vi "WT-Logger.vi"() -> ()   [LabVIEW 2017]
uses:
  <vilib>/Utility/file.llb/Write Delimited Spreadsheet (string).vi
  <vilib>/Utility/file.llb/Write Delimited Spreadsheet (DBL).vi
panel:
  out "Heart Beat":bool
  in  "File Output?":bool
  in  "Log_Data":bool
  out "MWTP":dbl(graph)
  out "LATP":dbl(graph)
  out "LATT":dbl(graph)
  out "LATD":dbl(graph)
  out "MWTV":dbl(graph)
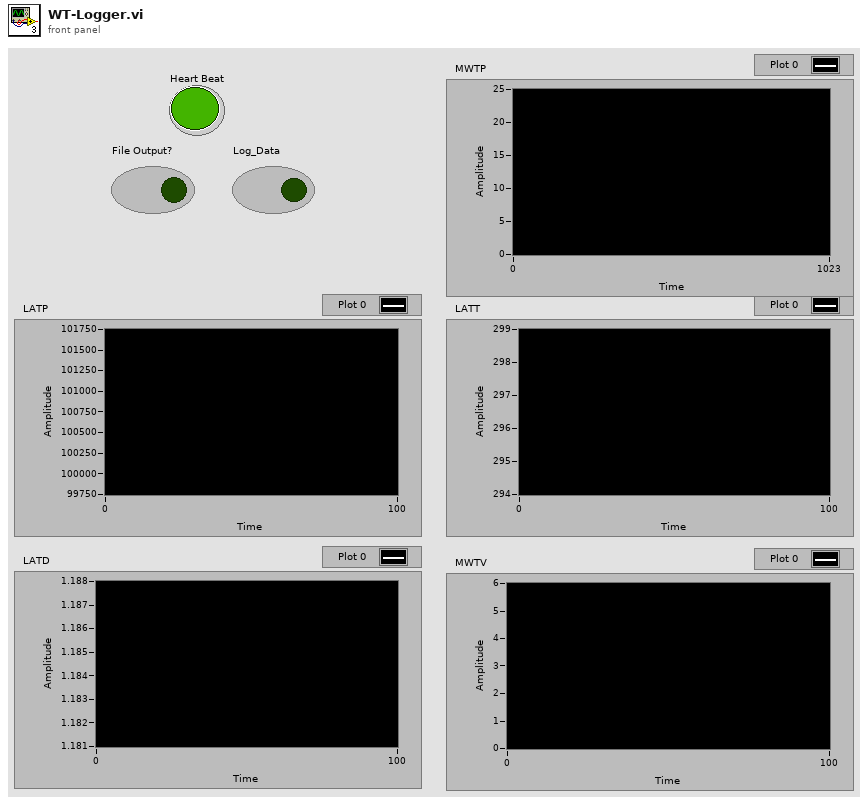
[diagram p1: front panel]
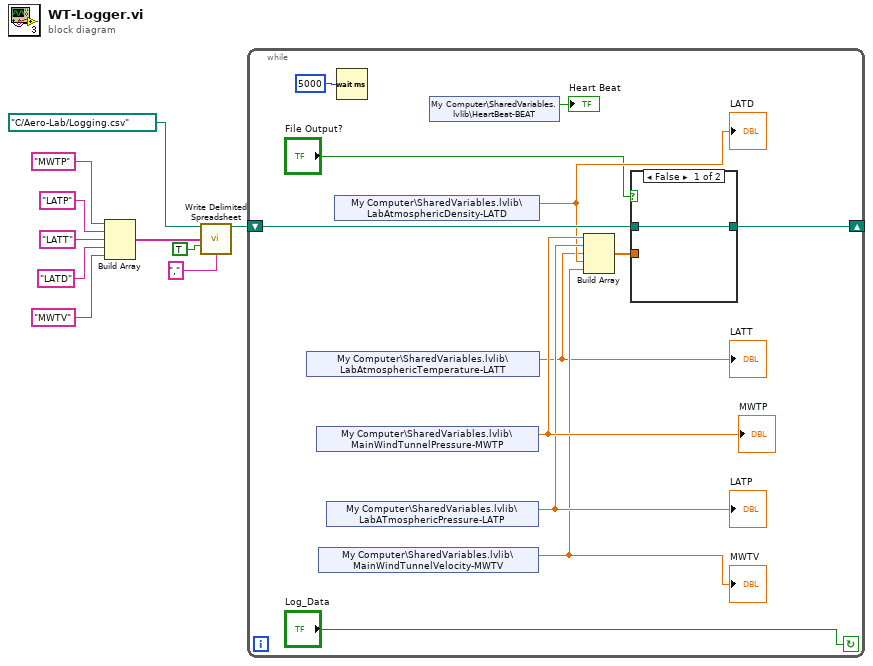
[diagram p0: block diagram]
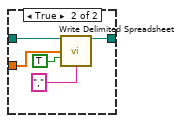
[diagram p2: hidden frame]
diagram:
  n1 = Build Array("MWTP", "LATP", "LATT", "LATD", "MWTV") -> (w4:string[])
  n2 = call-poly <vilib>:"Write Delimited Spreadsheet.vi"("file path (dialog if empty)"=path "C:/Aero-Lab/Logging.csv", "1D data"=w4, "append to file? (new file:F)"=TRUE, "delimiter (\\t)"="," ("delimiter (\\t)")) -> ("new file path (Not A Path if cancelled)"=w10:path)  [unwired: 10 in, 1 out]
  n3 = while {
    shift-right: [w20] -> _
    shift-left: w10 -> [w19]
    stop <- "Log_Data" continue-if-true
    n4 = shared-variable "My Computer\\SharedVariables.lvlib\\LabAtmosphericTemperature-LATT"() -> (w13:dbl)  [unwired: 1 in, 1 out]
    "LATT" <- w13
    n5 = shared-variable "My Computer\\SharedVariables.lvlib\\MainWindTunnelPressure-MWTP"() -> (w17:dbl)  [unwired: 1 in, 1 out]
    "MWTP" <- w17
    n6 = shared-variable "My Computer\\SharedVariables.lvlib\\MainWindTunnelVelocity-MWTV"() -> (w14:dbl)  [unwired: 1 in, 1 out]
    "MWTV" <- w14
    n7 = shared-variable "My Computer\\SharedVariables.lvlib\\LabATmosphericPressure-LATP"() -> (w16:dbl)  [unwired: 1 in, 1 out]
    "LATP" <- w16
    n8 = shared-variable "My Computer\\SharedVariables.lvlib\\LabAtmosphericDensity-LATD"() -> (w15:dbl)  [unwired: 1 in, 1 out]
    "LATD" <- w15
    n9 = Wait (ms)(milliseconds to wait=u32 5000 ("millisecond timer value")) -> ()  [unwired: 1 out]
    n10 = shared-variable "My Computer\\SharedVariables.lvlib\\HeartBeat-BEAT"() -> (→"Heart Beat":bool)  [unwired: 1 in, 1 out]
    n11 = Build Array(w17, w16, w13, w15, w14) -> (w18:dbl[])
    n12 = case shown="False" "File Output?" {
      tunnel: [w23 w26] -> w20
      tunnel: w19 -> [w23 w25]
      tunnel: w18 -> [_ w24]
      frame False {
      }
      frame True {
        n13 = call-poly <vilib>:"Write Delimited Spreadsheet.vi"("file path (dialog if empty)"=w25, "1D data"=w24, "append to file? (new file:F)"=TRUE, "delimiter (\\t)"="," ("delimiter (\\t)")) -> ("new file path (Not A Path if cancelled)"=w26:path)  [unwired: 10 in, 1 out]
      }
    }
  }
